vi "in_spline system y2.vi"(10 "X":dbl[](array[numeric]), 11 "Y":dbl[](array[numeric])) -> (2 "b":dbl[](array[numeric]), 3 "A":dbl[][](array[numeric]))   [LabVIEW 2020, in "NI_Gmath.lvlib"]
uses:
  NI_Gmath.lvlib
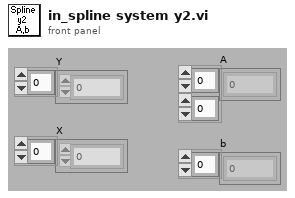
[diagram p1: front panel]
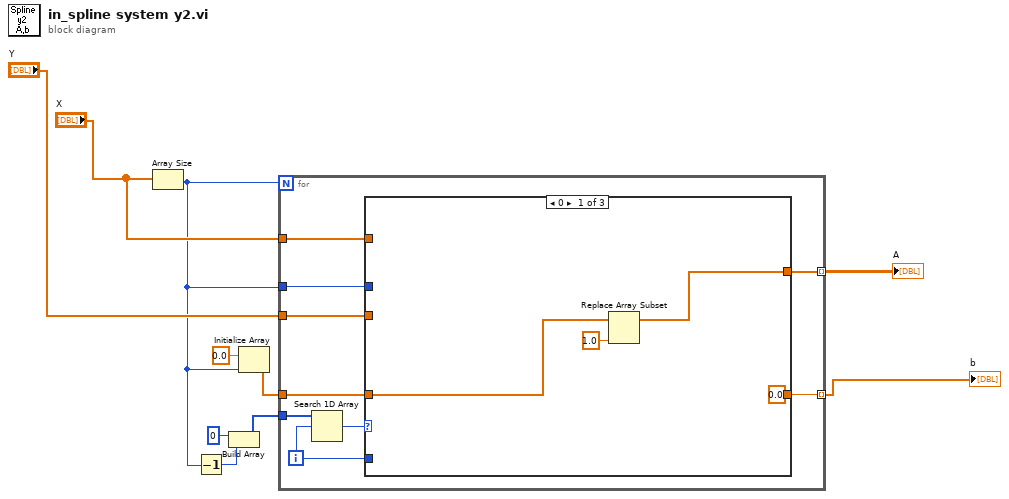
[diagram p0: block diagram]
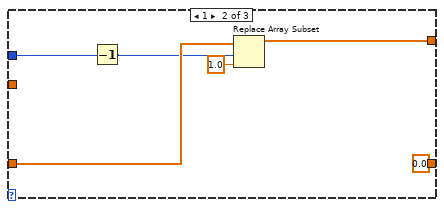
[diagram p2: hidden frame]
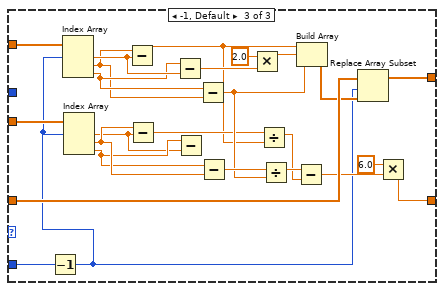
[diagram p3: hidden frame]
diagram:
  n1 = Array Size(array="X") -> (size(s)=w6:i32)
  n2 = Decrement(x=w6) -> (x-1=w4:i32)
  n3 = Build Array(0 ("element"), w4) -> (w5:i32[])
  n4 = Initialize Array(0.0 ("element"), w6) -> (w2:dbl[])
  n5 = for {
    N: w6 -> [_]
    tunnel: "X" -> [w19]
    tunnel: "Y" -> [w18]
    tunnel: w2 -> [w17]
    tunnel: [w16] -> w7 mode=indexing
    tunnel: w5 -> [w15]
    tunnel: [w12] -> w8 mode=indexing
    tunnel: w6 -> [w11]
    i -> [w13]
    n6 = Search 1D Array(1D array=w15, element=w13) -> (index of element=w14:i32)  [unwired: 1 in]
    n7 = case shown="0" w14 {
      tunnel: w19 -> [_ _ w54]
      tunnel: w18 -> [_ _ w47]
      tunnel: w17 -> [w22 w26 w44]
      tunnel: w13 -> [_ _ w31]
      tunnel: [w20 w27 w41] -> w16
      tunnel: [0.0 0.0 w33] -> w12
      tunnel: w11 -> [_ w25 _]
      frame 0 {
        n8 = Replace Array Subset(array=w22, new element=1.0 ("new element/subarray")) -> (w20:dbl[])  [unwired: 1 in]
      }
      frame 1 {
        n9 = Decrement(x=w25) -> (x-1=w24:i32)
        n10 = Replace Array Subset(array=w26, new element=1.0 ("new element/subarray"), index=w24) -> (w27:dbl[])
      }
      frame -1, Default {
        n11 = Decrement(x=w31) -> (x-1=w30:i32)
        n12 = Index Array(array=w54, index #1=w30) -> (element #1=w53:dbl, element #2=w51:dbl, element #3=w52:dbl)  [unwired: 2 in]
        n13 = Index Array(array=w47, index #1=w30) -> (element #1=w48:dbl, element #2=w50:dbl, element #3=w49:dbl)  [unwired: 2 in]
        n14 = Subtract(x=w51, y=w53) -> (x-y=w32:dbl)
        n15 = Subtract(x=w50, y=w48) -> (x-y=w37:dbl)
        n16 = Subtract(x=w52, y=w53) -> (x-y=w46:dbl)
        n17 = Subtract(x=w49, y=w48) -> ()  [unwired: 1 out]
        n18 = Subtract(x=w52, y=w51) -> (x-y=w39:dbl)
        n19 = Subtract(x=w49, y=w50) -> (x-y=w40:dbl)
        n20 = Multiply(x=2.0, y=w46) -> (x*y=w43:dbl)
        n21 = Divide(x=w37, y=w32) -> (x/y=w36:dbl)
        n22 = Divide(x=w40, y=w39) -> (x/y=w38:dbl)
        n23 = Subtract(x=w38, y=w36) -> (x-y=w34:dbl)
        n24 = Build Array(w32, w43, w39) -> (w42:dbl[])
        n25 = Replace Array Subset(array=w44, new element=w42, index=w30) -> (w41:dbl[])
        n26 = Multiply(x=6.0, y=w34) -> (x*y=w33:dbl)
      }
    }
  }
  "b" <- w8
  "A" <- w7
